vi "Compute 1D Index__ogtk.vi"(1 "Size(s)":u32[](array[numeric]), 2 "Indices":u32[](array[numeric])) -> (0 "1D Index":i32)   [LabVIEW 2023, in "openg_variant.lvlib"]
doc: "Returns the 1D index incorresponding to the element of a MultiD array at given indices."
uses:
  openg_variant.lvlib
panel:
  # "[OpenG VI Tags] ***Do Not Remove***"
  # "Compute 1D Index.vi\n\nReturns the 1D index incorresponding to the element of a MultiD array at given i\n\nPlease visit http://www.OpenG.org to learn about the\nOpen Source LabVIEW software movement.\n\nNOTICE -- YOU MUST LEAVE THIS NOTICE IN PLACE.  PER THE TERMS OF THE LICENSE BELOW, YOU MAY SUBLICENSE THIS SOFTWARE \nIN ANY WAY THAT DOES NOT CONFLICT WITH THIS LICENSE.\n\n### BSD License (http://www.opensource.org/licenses/bsd-license.php) Begin ###\n \nCopyright (c) 2002, Jean-Pierre Drolet <drolet_jp@hotmail.com>\nCopyright (c) 2002-2006, Jim Kring <jim@jimkring.com>\n\nAll rights reserved.\n\nRedistribution and use in source and binary forms, with or without modification, are permitted provided that the following conditions are met:\n\n    * Redistributions of source code must retain the above copyright notice, this list of conditions and the following disclaimer.\n    * Redistributions in binary form must reproduce the above copyright notice, this list of conditions and the following disclaimer in the \n       documentation and/or other materials provided with the distribution.\n    * Neither the name of SciWare, James Kring, Inc., nor the names of its contributors may be used to endorse or promote products derived \n       from this software without specific prior written permission.\n\nTHIS SOFTWARE IS PROVIDED BY THE COPYRIGHT HOLDERS AND CONTRIBUTORS \"AS IS\" AND ANY EXPRESS OR IMPLIED WARRANTIES, \nINCLUDING, BUT NOT LIMITED TO, THE IMPLIED WARRANTIES OF MERCHANTABILITY AND FITNESS FOR A PARTICULAR PURPOSE ARE \nDISCLAIMED. IN NO EVENT SHALL THE COPYRIGHT OWNER OR CONTRIBUTORS BE LIABLE FOR ANY DIRECT, INDIRECT, INCIDENTAL,\n SPECIAL, EXEMPLARY, OR CONSEQUENTIAL DAMAGES (INCLUDING, BUT NOT LIMITED TO, PROCUREMENT OF SUBSTITUTE GOODS OR \nSERVICES; LOSS OF USE, DATA, OR PROFITS; OR BUSINESS INTERRUPTION) HOWEVER CAUSED AND ON ANY THEORY OF LIABILITY, \nWHETHER IN CONTRACT, STRICT LIABILITY, OR TORT (INCLUDING NEGLIGENCE OR OTHERWISE) ARISING IN ANY WAY OUT OF THE USE \nOF THIS SOFTWARE, EVEN IF ADVISED OF THE POSSIBILITY OF SUCH DAMAGE.\n\n### BSD License End ###"
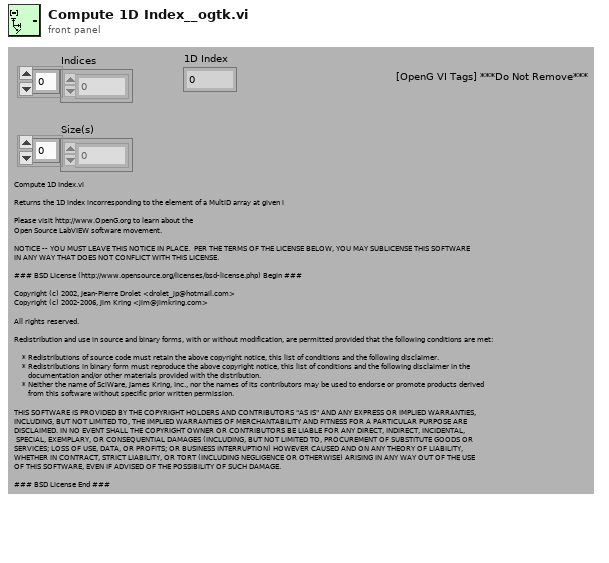
[diagram p1: front panel]
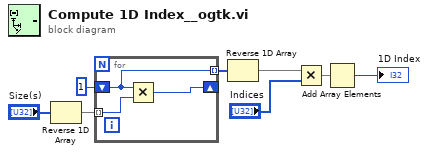
[diagram p0: block diagram]
diagram:
  n1 = Reverse 1D Array(array="Size(s)") -> (reversed array=w3:u32[])
  n2 = for {
    shift-right: [w10] -> _
    shift-left: 1 ("Index") -> [w9]
    tunnel: w3 -> [w11] mode=indexing
    tunnel: [w9] -> w2 mode=indexing
    n3 = Multiply(x=w9, y=w11) -> (x*y=w10:u32)
  }
  n4 = Reverse 1D Array(array=w2) -> (reversed array=w1:u32[])
  n5 = Multiply(x=w1, y="Indices") -> (x*y=w7:u32[])
  n6 = Add Array Elements(numeric array=w7) -> (sum=→"1D Index":u32)
